vi "Get Installed Software 1.0.vi"   [LabVIEW 2012, in "nisyscfg.lvlib"]
doc: "Retrieves a list of software installed on the RT system."
uses:
  <vilib>/nisyscfg/nisyscfg.lvlib
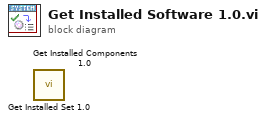
[diagram p0: block diagram]
diagram:
  n1 = call <vilib>:"Get Installed Set 1.0.vi"() -> ()  [unwired: 9 in, 3 out]
  n2 = call <vilib>:"Get Installed Components 1.0.vi"() -> ()  [unwired: 9 in, 3 out]
